vi "DataLog Read Log Strings.vi"(0 "tag log directory":path, 5 "offsets (use points)":dbl[](array[numeric]), 7 "points (use offsets)":T1[](array[typedef]) {"value" format="%.3e"; "time" format="%<%H:%M:%S%2u\n%Y/%m/%d>T"}, 11 "error in (no error)":errorcluster) -> (4 "dup tag log directory":path, 6 "times":dbl[](array[numeric]) format="%<%H:%M:%S%2u\n%Y/%m/%d>T", 8 "strings":string[](array[string]), 15 "error out":errorcluster)   [LabVIEW 2012]
doc: "Read the strings at the specified byte offsets from the strings file of a string tag log. These offsets are stored as the values of the tag's point. Consequently, to use this function, you must pass a range of points read from the tag's log or their offset values."
uses:
  typedefs/clusters/t_DataLog Point.ctl
  private/glb_DataLog Runtime Parameterisation.vi
  private/glb_DataLog MCVD.vi
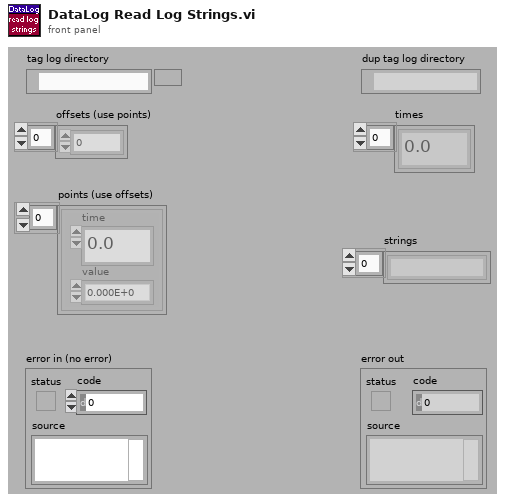
[diagram p1: front panel]
types:
  T1 = typedef "t_DataLog Point.ctl" = cluster{"time":dbl, "value":dbl}
  T2 = enum16{"read/write", "read-only", "write-only", "write-only (truncate)"}
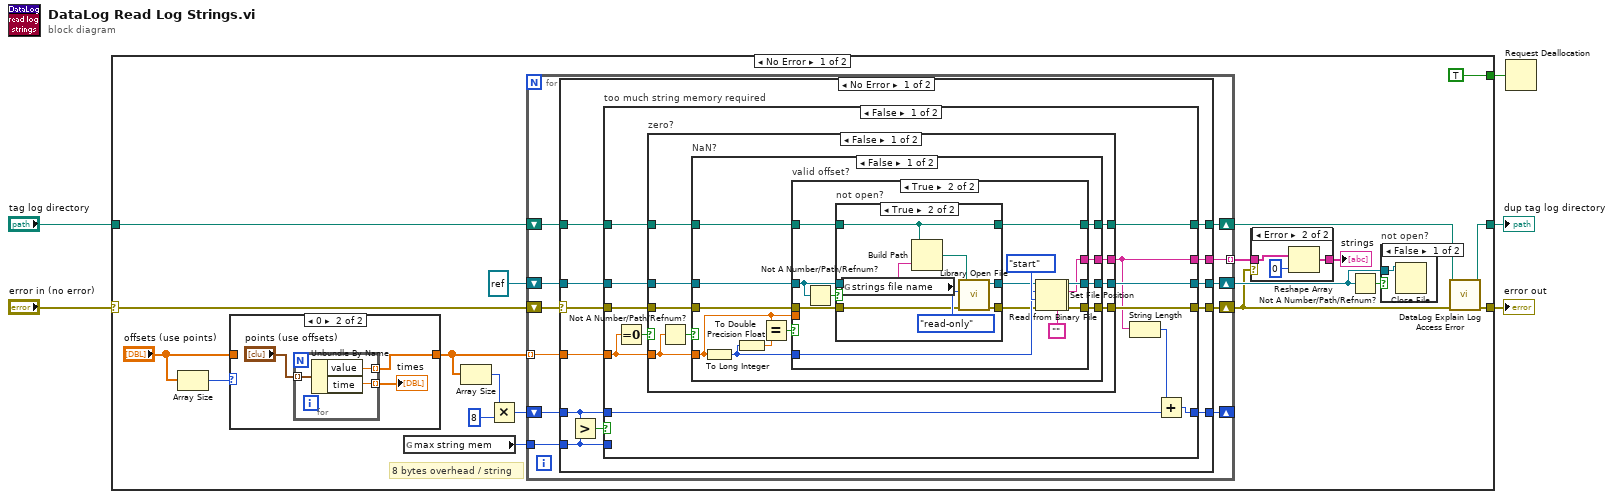
[diagram p0: block diagram]
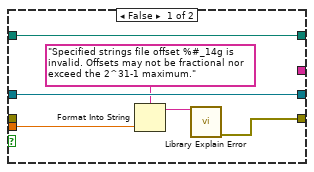
[diagram p5: hidden frame]
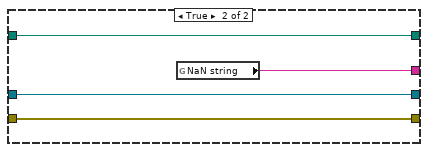
[diagram p7: hidden frame]
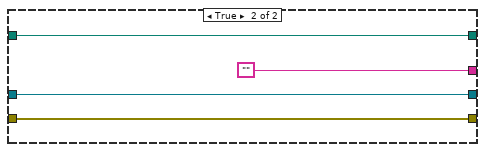
[diagram p8: hidden frame]
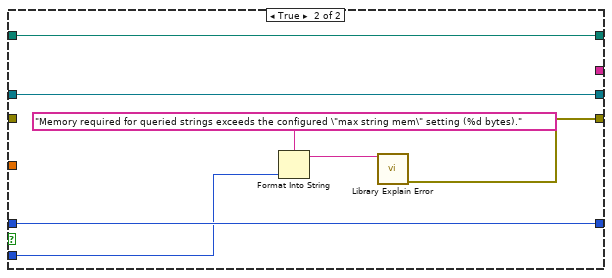
[diagram p9: hidden frame]
diagram:
  n1 = case shown="No Error" "error in (no error)" {
    selector: "error in (no error)" -> [w16 w143]
    tunnel: [w24 w143] -> w5
    tunnel: "tag log directory" -> [w18 w142]
    tunnel: [w23 w142] -> w2
    tunnel: [TRUE _] -> w1
    frame No Error {
      # "8 bytes overhead / string"
      n2 = Array Size(array="offsets (use points)") -> (size(s)=w15:i32)
      n3 = case shown="0" w15 {
        tunnel: "offsets (use points)" -> [w29 _]
        tunnel: [w29 w30] -> w11
        frame Default {
        }
        frame 0 {
          n4 = for {
            tunnel: "points (use offsets)" -> [w35] mode=indexing
            tunnel: [w34] -> w31 mode=indexing
            tunnel: [w33] -> w30 mode=indexing
            n5 = Unbundle By Name(w35) -> ("value"=w33:dbl, "time"=w34:dbl)
          }
          "times" <- w31
        }
      }
      n6 = global read "glb_DataLog Runtime Parameterisation.vi" "max string mem"() -> (w7:i32)
      n7 = Array Size(array=w11) -> (size(s)=w10:i32)
      n8 = Multiply(x=w10, y=8) -> (x*y=w8:i32)
      n9 = for {
        shift-right: [w47] -> w19
        shift-left: refnum<file> refnum ("refnum") -> [w45]
        shift-right: [w46] -> w12
        shift-left: w16 -> [w43]
        tunnel: [w44] -> w22 mode=indexing
        shift-right: [w41] -> w17
        shift-left: w18 -> [w42]
        tunnel: w11 -> [w40] mode=indexing
        shift-right: [w38] -> _
        shift-left: w8 -> [w39]
        tunnel: w7 -> [w37]
        n10 = case shown="No Error" w43 {
          selector: w43 -> [w56 w140]
          tunnel: [w59 w141] -> w47
          tunnel: [w58 w140] -> w46
          tunnel: w45 -> [w57 w141]
          tunnel: w40 -> [w55 _]
          tunnel: [w52 _] -> w44
          tunnel: w42 -> [w54 w139]
          tunnel: [w53 w139] -> w41
          tunnel: w39 -> [w50 w138]
          tunnel: [w51 w138] -> w38
          tunnel: w37 -> [w48 _]
          frame No Error {
            n11 = Greater?(x=w50, y=w48) -> (0:w49:bool)
            n12 = case "too much string memory required" shown="False" w49 {
              tunnel: [w71 w135] -> w59
              tunnel: [w70 w131] -> w58
              tunnel: w57 -> [w69 w135]
              tunnel: w56 -> [w68 _]
              tunnel: w55 -> [w66 _]
              tunnel: w54 -> [w65 w136]
              tunnel: [w64 w136] -> w53
              tunnel: w50 -> [w63 w137]
              tunnel: [w62 _] -> w52
              tunnel: [w60 w137] -> w51
              tunnel: w48 -> [_ w134]
              frame False {
                n13 = Equal To 0?(x=w66) -> (x = 0?=w67:bool)
                n14 = case "zero?" shown="False" w67 {
                  tunnel: [w80 w129] -> w71
                  tunnel: [w79 w128] -> w70
                  tunnel: w69 -> [w78 w129]
                  tunnel: w66 -> [w75 _]
                  tunnel: [w77 ""] -> w62
                  tunnel: w68 -> [w76 w128]
                  tunnel: w65 -> [w73 w127]
                  tunnel: [w72 w127] -> w64
                  frame False {
                    n15 = Not A Number/Path/Refnum?(number/path/refnum=w75) -> (NaN/Path/Refnum?=w74:bool)
                    n16 = case "NaN?" shown="False" w74 {
                      tunnel: [w91 w126] -> w80
                      tunnel: [w90 w125] -> w79
                      tunnel: w78 -> [w88 w126]
                      tunnel: w75 -> [w81 _]
                      tunnel: [w89 w123] -> w77
                      tunnel: w76 -> [w87 w125]
                      tunnel: w73 -> [w86 w124]
                      tunnel: [w85 w124] -> w72
                      frame False {
                        n17 = To Long Integer(number=w81) -> (32bit integer=w84:i32)
                        n18 = To Double Precision Float(number=w84) -> (double precision float=w83:dbl)
                        n19 = Equal?(x=w81, y=w83) -> (x = y?=w82:bool)
                        n20 = case "valid offset?" shown="True" w82 {
                          tunnel: [w96 w111] -> w91
                          tunnel: [w92 w110] -> w90
                          tunnel: w84 -> [_ w108]
                          tunnel: [_ w107] -> w89
                          tunnel: w88 -> [w96 w105]
                          tunnel: w87 -> [_ w104]
                          tunnel: w86 -> [w97 w101]
                          tunnel: [w97 w100] -> w85
                          tunnel: w81 -> [w94 _]
                          frame False {
                            n21 = Format Into String(format string="Specified strings file offset %#_14g is invalid. Offsets may not be fractional nor exceed the 2^31-1 maximum.", w94) -> (resulting string=w95:string)  [unwired: 2 in, 1 out]
                            n22 = call "Library Explain Error.vi"("explanation prefix (none)"=w95) -> ("explained error"=w92:errorcluster)  [unwired: 14 in]
                          }
                          frame True {
                            n23 = Not A Number/Path/Refnum?(number/path/refnum=w105) -> (NaN/Path/Refnum?=w106:bool)
                            n24 = case "not open?" shown="True" w106 {
                              tunnel: w105 -> [w115 _]
                              tunnel: w104 -> [w114 w121]
                              tunnel: [w114 w120] -> w103
                              tunnel: [w115 w119] -> w102
                              tunnel: w101 -> [w113 w116]
                              tunnel: [w113 w116] -> w100
                              frame False {
                              }
                              frame True {
                                n25 = global read "glb_DataLog MCVD.vi" "strings file name"() -> (w118:string)
                                n26 = Build Path(base path=w116, name or relative path=w118) -> (appended path=w117:path)
                                n27 = call "Library Open File.vi"("error in (no error)"=w121, "open mode (read/write)"=T2."read-only" ("open mode (0)"), "file path"=w117) -> ("error out"=w120:errorcluster, "refnum"=w119:refnum<file>)  [unwired: 3 in]
                              }
                            }
                            n28 = Set File Position(offset (in bytes) (0)=w108, refnum=w102, from (0:start)=enum16{"start", "end", "current"}."start" ("pos mode (0:2)"), error in=w103) -> (refnum out=w99:refnum<file>, error out=w98:errorcluster)
                            n29 = Read from Binary File(5:"", 8:w98, 11:w99) -> (0:w110:errorcluster, 2:w107:string, 3:w111:refnum<file>)  [unwired: 3 in, 1 out]
                          }
                        }
                      }
                      frame True {
                        n30 = global read "glb_DataLog MCVD.vi" "NaN string"() -> (w123:string)
                      }
                    }
                  }
                  frame True {
                  }
                }
                n31 = String Length(string=w62) -> (length=w61:i32)
                n32 = Add(x=w61, y=w63) -> (x+y=w60:i32)
              }
              frame True {
                n33 = Format Into String(format string="Memory required for queried strings exceeds the configured \"max string mem\" setting (%d bytes).", w134) -> (resulting string=w132:string)  [unwired: 2 in, 1 out]
                n34 = call "Library Explain Error.vi"("explanation prefix (none)"=w132) -> ("explained error"=w131:errorcluster)  [unwired: 14 in]
              }
            }
          }
          frame Error {
          }
        }
      }
      n35 = case shown="Error" w12 {
        tunnel: w22 -> [w25 w28]
        tunnel: [w25 w27] -> w13
        frame No Error {
        }
        frame Error {
          n36 = Reshape Array(w28, 0 ("dimension size")) -> (w27:string[])
        }
      }
      "strings" <- w13
      n37 = Not A Number/Path/Refnum?(number/path/refnum=w19) -> (NaN/Path/Refnum?=w20:bool)
      n38 = case "not open?" shown="False" w20 {
        tunnel: w19 -> [w36 _]
        frame False {
          n39 = Close File(refnum=w36) -> ()  [unwired: 1 in, 2 out]
        }
        frame True {
        }
      }
      n40 = call "DataLog Explain Log Access Error.vi"("tag log directory"=w17, "error in"=w12) -> ("dup tag log directory"=w23:path, "error out"=w24:errorcluster)  [unwired: 12 in]
    }
    frame Error {
    }
  }
  "error out" <- w5
  "dup tag log directory" <- w2
  n41 = Request Deallocation(w1) -> ()
